vi "Initialize.vi"(7 "not in use":string="Setpoint.ch%d.SP", 8 "error in":errorcluster, 9 "Number of Channels":u32=1, 10 "Instance Name":string, 11 "Power Supply In":refnum<class "Power Supply.lvclass">) -> (0 "error out":errorcluster, 2 "Channel":T1[](array[typedef]), 3 "Power Supply Out":refnum<class "Power Supply.lvclass">)   [LabVIEW 2023, in "Power Supply.lvclass"]
uses:
  Power Supply.lvclass
  Low Level Capabilities/Current/Current Setpoint/Current Setpoint.lvclass
  Low Level Capabilities/Voltage/Voltage Actual Value/Voltage Actual Value.lvclass
  Low Level Capabilities/Voltage/Voltage Setpoint/Voltage Setpoint.lvclass
  Low Level Capabilities/Current/Current Actual Value/Current Actual Value.lvclass
  Low Level Capabilities/Current/Current Limit/Current Limit.lvclass
  Low Level Capabilities/Error Channels/Error Channels.lvclass
  Low Level Capabilities/Control Mode/Control Mode.lvclass
  Low Level Capabilities/Voltage/Voltage Limit/Voltage Limit.lvclass
  Low Level Capabilities/Power/Power Limit/Power Limit.lvclass
  Low Level Capabilities/Power/Power Actual Value/Power Actual Value.lvclass
  Low Level Capabilities/Power/Power Setpoint/Power Setpoint.lvclass
  Low Level Capabilities/Error/Error.lvclass
  Low Level Capabilities/OnOff/OnOff.lvclass
  Low Level Capabilities/Output Enable/Output Enable.lvclass
  Low Level Capabilities/Power/Power Gradient/Power Gradient.lvclass
  Low Level Capabilities/Voltage/Voltage Gradient/Voltage Gradient.lvclass
  Low Level Capabilities/Current/Current Gradient/Current Gradient.lvclass
  Utilities/Channel.ctl
  Utilities/Utilities.lvlib
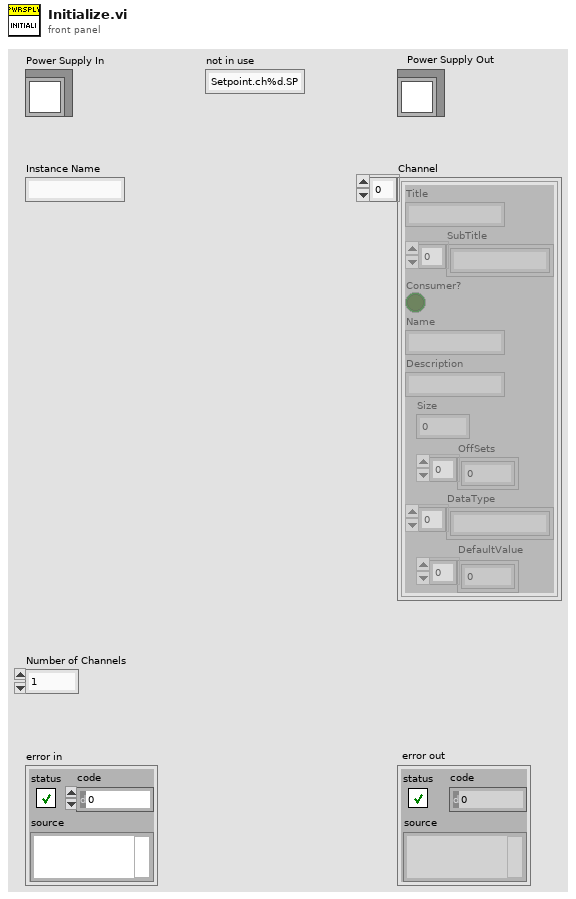
[diagram p1: front panel]
types:
  T1 = typedef "Utilities.lvlib/Channel.ctl" = cluster{"Title":string, "SubTitle":string[], "Consumer?":bool, "Name":string, "Description":string, "Size":i32, "OffSets":i32[], "DataType":string[], "DefaultValue":dbl[]}
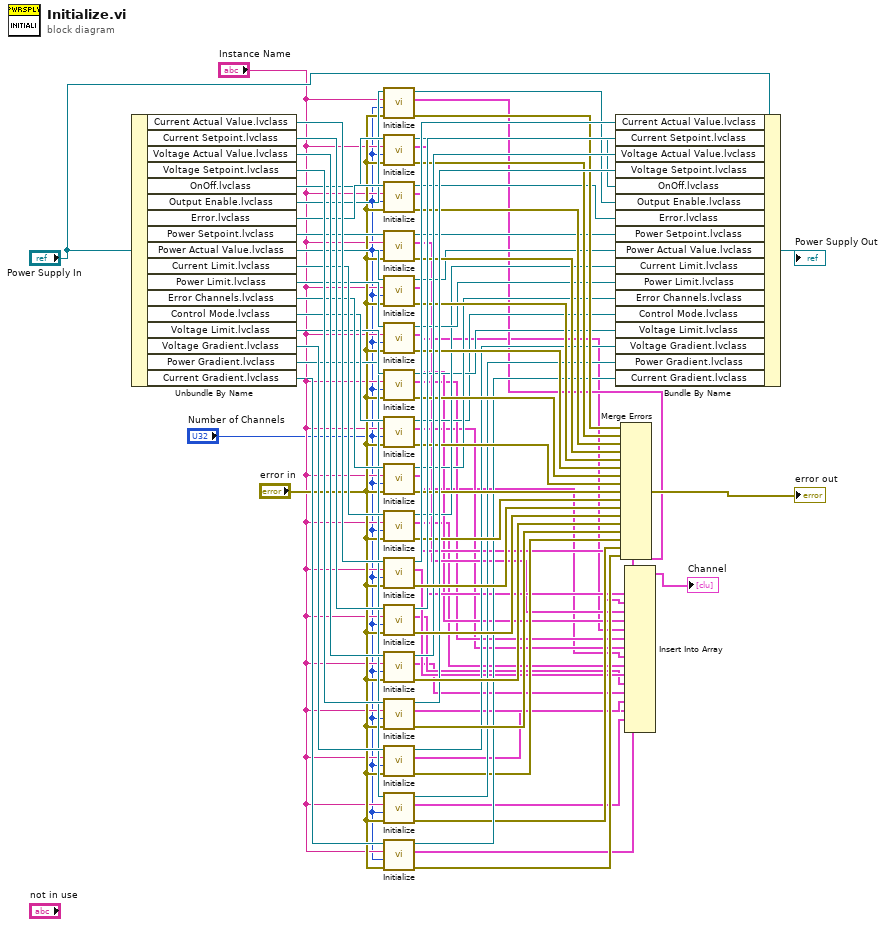
[diagram p0: block diagram]
diagram:
  n1 = Unbundle By Name("Power Supply In") -> ("Current Actual Value.lvclass"=w67:refnum<class "Current Actual Value.lvclass">, "Current Setpoint.lvclass"=w66:refnum<class "Current Setpoint.lvclass">, "Voltage Actual Value.lvclass"=w64:refnum<class "Voltage Actual Value.lvclass">, "Voltage Setpoint.lvclass"=w63:refnum<class "Voltage Setpoint.lvclass">, "OnOff.lvclass"=w44:refnum<class "OnOff.lvclass">, "Output Enable.lvclass"=w41:refnum<class "Output Enable.lvclass">, "Error.lvclass"=w45:refnum<class "Error.lvclass">, "Power Setpoint.lvclass"=w47:refnum<class "Power Setpoint.lvclass">, "Power Actual Value.lvclass"=w50:refnum<class "Power Actual Value.lvclass">, "Current Limit.lvclass"=w60:refnum<class "Current Limit.lvclass">, "Power Limit.lvclass"=w52:refnum<class "Power Limit.lvclass">, "Error Channels.lvclass"=w58:refnum<class "Error Channels.lvclass">, "Control Mode.lvclass"=w56:refnum<class "Control Mode.lvclass">, "Voltage Limit.lvclass"=w53:refnum<class "Voltage Limit.lvclass">, "Voltage Gradient.lvclass"=w27:refnum<class "Voltage Gradient.lvclass">, "Power Gradient.lvclass"=w26:refnum<class "Power Gradient.lvclass">, "Current Gradient.lvclass"=w25:refnum<class "Current Gradient.lvclass">)
  n2 = call-dynamic "Initialize.vi"("error in"="error in", "Number of Channels"="Number of Channels", "Instance Name"="Instance Name", "Output Enable in"=w41) -> ("error out"=w42:errorcluster, "Channel"=w18:T1[], "Output Enable out"=w39:refnum<class "Output Enable.lvclass">)  [unwired: 5 in]
  n3 = call-dynamic "Initialize.vi"("error in"="error in", "Number of Channels"="Number of Channels", "Instance Name"="Instance Name", "OnOff in"=w44) -> ("error out"=w43:errorcluster, "Channel"=w17:T1[], "OnOff out"=w40:refnum<class "OnOff.lvclass">)  [unwired: 5 in]
  n4 = call-dynamic "Initialize.vi"("error in"="error in", "Number of Channels"="Number of Channels", "Instance Name"="Instance Name", "Error in"=w45) -> ("error out"=w46:errorcluster, "Channel"=w16:T1[], "Error out"=w38:refnum<class "Error.lvclass">)  [unwired: 5 in]
  n5 = call-dynamic "Initialize.vi"("error in"="error in", "Number of Channels"="Number of Channels", "Instance Name"="Instance Name", "Power Setpoint in"=w47) -> ("error out"=w48:errorcluster, "Channel"=w15:T1[], "Power Setpoint out"=w37:refnum<class "Power Setpoint.lvclass">)  [unwired: 5 in]
  n6 = call-dynamic "Initialize.vi"("error in"="error in", "Number of Channels"="Number of Channels", "Instance Name"="Instance Name", "Power Actual Value in"=w50) -> ("error out"=w49:errorcluster, "Channel"=w14:T1[], "Power Actual Value out"=w36:refnum<class "Power Actual Value.lvclass">)  [unwired: 5 in]
  n7 = call-dynamic "Initialize.vi"("error in"="error in", "Number of Channels"="Number of Channels", "Instance Name"="Instance Name", "Power Limit in"=w52) -> ("error out"=w51:errorcluster, "Channel"=w13:T1[], "Power Limit out"=w35:refnum<class "Power Limit.lvclass">)  [unwired: 5 in]
  n8 = call-dynamic "Initialize.vi"("error in"="error in", "Number of Channels"="Number of Channels", "Instance Name"="Instance Name", "Voltage Limit in"=w53) -> ("error out"=w54:errorcluster, "Channel"=w12:T1[], "Voltage Limit out"=w32:refnum<class "Voltage Limit.lvclass">)  [unwired: 5 in]
  n9 = call-dynamic "Initialize.vi"("error in"="error in", "Number of Channels"="Number of Channels", "Instance Name"="Instance Name", "Control Mode in"=w56) -> ("error out"=w55:errorcluster, "Channel"=w11:T1[], "Control Mode out"=w31:refnum<class "Control Mode.lvclass">)  [unwired: 5 in]
  n10 = call-dynamic "Initialize.vi"("error in"="error in", "Number of Channels"="Number of Channels", "Instance Name"="Instance Name", "Error Channels in"=w58) -> ("error out"=w57:errorcluster, "Channel"=w10:T1[], "Error Channels out"=w33:refnum<class "Error Channels.lvclass">)  [unwired: 5 in]
  n11 = call-dynamic "Initialize.vi"("error in"="error in", "Number of Channels"="Number of Channels", "Instance Name"="Instance Name", "Current Limit in"=w60) -> ("error out"=w59:errorcluster, "Channel"=w9:T1[], "Current Limit out"=w34:refnum<class "Current Limit.lvclass">)  [unwired: 5 in]
  n12 = call-dynamic "Initialize.vi"("error in"="error in", "Number of Channels"="Number of Channels", "Instance Name"="Instance Name", "Current Actual Value in"=w67) -> ("error out"=w74:errorcluster, "Channel"=w8:T1[], "Current Actual Value out"=w68:refnum<class "Current Actual Value.lvclass">)  [unwired: 5 in]
  n13 = call-dynamic "Initialize.vi"("error in"="error in", "Number of Channels"="Number of Channels", "Instance Name"="Instance Name", "Current Setpoint in"=w66) -> ("error out"=w75:errorcluster, "Channel"=w7:T1[], "Current Setpoint out"=w65:refnum<class "Current Setpoint.lvclass">)  [unwired: 5 in]
  n14 = call-dynamic "Initialize.vi"("error in"="error in", "Number of Channels"="Number of Channels", "Instance Name"="Instance Name", "Voltage Actual Value in"=w64) -> ("error out"=w73:errorcluster, "Channel"=w6:T1[], "Voltage Actual Value out"=w62:refnum<class "Voltage Actual Value.lvclass">)  [unwired: 5 in]
  n15 = call-dynamic "Initialize.vi"("error in"="error in", "Number of Channels"="Number of Channels", "Instance Name"="Instance Name", "Voltage Setpoint in"=w63) -> ("error out"=w72:errorcluster, "Channel"=w5:T1[], "Voltage Setpoint out"=w61:refnum<class "Voltage Setpoint.lvclass">)  [unwired: 5 in]
  n16 = call-dynamic "Initialize.vi"("error in"="error in", "Number of Channels"="Number of Channels", "Instance Name"="Instance Name", "Voltage Gradient in"=w27) -> ("error out"=w22:errorcluster, "Channel"=w4:T1[], "Voltage Gradient out"=w30:refnum<class "Voltage Gradient.lvclass">)  [unwired: 5 in]
  n17 = call-dynamic "Initialize.vi"("error in"="error in", "Number of Channels"="Number of Channels", "Instance Name"="Instance Name", "Power Gradient in"=w26) -> ("error out"=w20:errorcluster, "Channel"=w3:T1[], "Power Gradient out"=w29:refnum<class "Power Gradient.lvclass">)  [unwired: 5 in]
  n18 = call-dynamic "Initialize.vi"("error in"="error in", "Number of Channels"="Number of Channels", "Instance Name"="Instance Name", "Current Gradient in"=w25) -> ("error out"=w19:errorcluster, "Channel"=w2:T1[], "Current Gradient out"=w28:refnum<class "Current Gradient.lvclass">)  [unwired: 5 in]
  n19 = Bundle By Name(cluster="Power Supply In", "Current Actual Value.lvclass"=w68, "Current Setpoint.lvclass"=w65, "Voltage Actual Value.lvclass"=w62, "Voltage Setpoint.lvclass"=w61, "OnOff.lvclass"=w40, "Output Enable.lvclass"=w39, "Error.lvclass"=w38, "Power Setpoint.lvclass"=w37, "Power Actual Value.lvclass"=w36, "Current Limit.lvclass"=w34, "Power Limit.lvclass"=w35, "Error Channels.lvclass"=w33, "Control Mode.lvclass"=w31, "Voltage Limit.lvclass"=w32, "Voltage Gradient.lvclass"=w30, "Power Gradient.lvclass"=w29, "Current Gradient.lvclass"=w28) -> (→"Power Supply Out":refnum<class "Power Supply.lvclass">)
  n20 = Merge Errors(w42, w43, w46, w48, w49, w51, w54, w55, w57, w59, w74, w75, w73, w72, w22, w20, w19) -> (→"error out":errorcluster)
  n21 = Insert Into Array(array=w18, new element #1=w17, new element #2=w16, new element #3=w15, new element #4=w14, new element #5=w13, new element #6=w12, new element #7=w11, new element #8=w10, new element #9=w9, new element #10=w8, new element #11=w7, new element #12=w6, new element #13=w5, new element #14=w4, new element #15=w3, new element #16=w2) -> (→"Channel":T1[])  [unwired: 1 in]
